vi "_Yoko_precision.vi"(6 "GPIB address (19)":string="2") -> (1 "String":string, 2 "Precision":i16, 3 "Regime":i16)   [LabVIEW 2013]
panel:
  out "String 2":string
  out "error out":errorcluster
  in  "error in (no error)":errorcluster
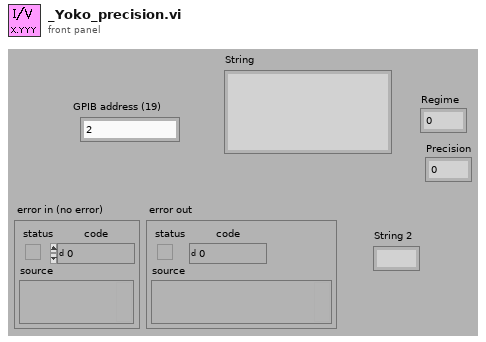
[diagram p1: front panel]
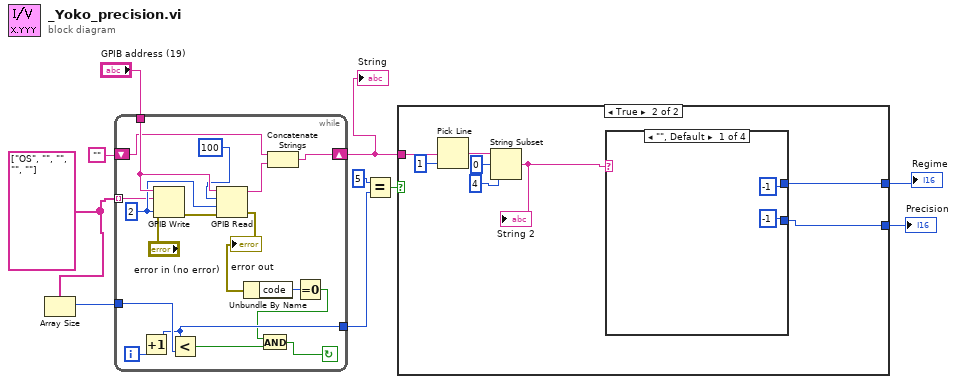
[diagram p0: block diagram]
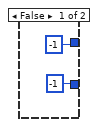
[diagram p2: hidden frame]
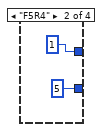
[diagram p3: hidden frame]
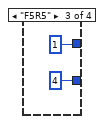
[diagram p4: hidden frame]
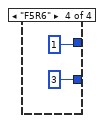
[diagram p5: hidden frame]
diagram:
  w9 = string[] ["OS", "", "", "", ""] ("Array")
  n1 = Array Size(array=w9) -> (size(s)=w8:i32)
  n2 = while {
    tunnel: "GPIB address (19)" -> [w27]
    tunnel: w9 -> [w18] mode=indexing
    shift-right: [w17] -> w4
    shift-left: "" -> [w19]
    tunnel: w8 -> [w16]
    tunnel: [w14] -> w5
    i -> [w15]
    stop <- w12 continue-if-true
    w24 = 2
    n3 = Increment(x=w15) -> (x+1=w14:i32)
    n4 = GPIB Write(0:w27, 1:w18, 2:w24, 3:"error in (no error)") -> (6:w25:errorcluster)  [unwired: 1 in, 1 out]
    n5 = Less?(x=w14, y=w16) -> (x < y?=w13:bool)
    n6 = GPIB Read(0:w27, 1:100, 2:w24, 3:w25) -> (5:w20:string, 7:w22:errorcluster)  [unwired: 1 in, 1 out]
    "error out" <- w22
    n7 = Unbundle By Name(w22) -> ("code"=w21:i32)
    n8 = Concatenate Strings(w19, w20) -> (w17:string)
    n9 = Equal To 0?(x=w21) -> (x = 0?=w11:bool)
    n10 = And(x=w11, y=w13) -> (x .and. y?=w12:bool)
  }
  "String" <- w4
  n11 = Equal?(x=5, y=w5) -> (x = y?=w7:bool)
  n12 = case shown="True" w7 {
    tunnel: w4 -> [_ w37]
    tunnel: [-1 w31] -> w3
    tunnel: [-1 w30] -> w2
    frame False {
    }
    frame True {
      n13 = Pick Line(multi-line string=w37, line index=1) -> (output string=w35:string)  [unwired: 1 in]
      n14 = String Subset(string=w35, offset (0)=0, length (rest)=4) -> (substring=w32:string)
      "String 2" <- w32
      n15 = case shown="\"\", Default" w32 {
        tunnel: [-1 1 1 1] -> w31
        tunnel: [-1 5 4 3] -> w30
        frame "", Default {
        }
        frame "F5R4" {
        }
        frame "F5R5" {
        }
        frame "F5R6" {
        }
      }
    }
  }
  "Regime" <- w3
  "Precision" <- w2
